vi "Load.vi"(0 "TxA in":T1, 1 "section (optional)":string, 5 "TxO in":T2, 7 "Tx in":T3, 9 "PxA in":T4, 12 "PxO in":T5, 13 "Px in":T6) -> (3 "Px out":T6, 4 "PxO out":T5, 6 "PxA out":T4, 8 "Tx out":T3, 10 "TxO out":T2, 14 "TxA out":T1)   [LabVIEW 2017, in "Konfiguracja.lvlib"]
uses:
  Libraries/Konfiguracja/Konfiguracja.lvlib
  <vilib>/Utility/config.llb/NI_LVConfig.lvlib
  Controls/TxA.ctl
  Controls/TxO.ctl
  Controls/Tx.ctl
  Controls/PxA.ctl
  Controls/Px0.ctl
  Controls/Px.ctl
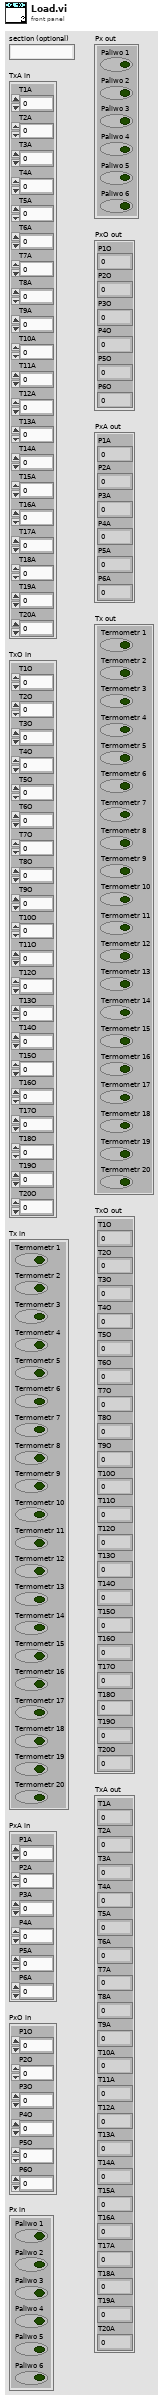
[diagram p1: front panel]
types:
  T1 = typedef "Konfiguracja.lvlib/TxA.ctl" = cluster{"T1A":dbl, "T2A":dbl, "T3A":dbl, "T4A":dbl, "T5A":dbl, "T6A":dbl, "T7A":dbl, "T8A":dbl, "T9A":dbl, "T10A":dbl, "T11A":dbl, "T12A":dbl, "T13A":dbl, "T14A":dbl, "T15A":dbl, "T16A":dbl, "T17A":dbl, "T18A":dbl, "T19A":dbl, "T20A":dbl}
  T2 = typedef "Konfiguracja.lvlib/TxO.ctl" = cluster{"T1O":dbl, "T2O":dbl, "T3O":dbl, "T4O":dbl, "T5O":dbl, "T6O":dbl, "T7O":dbl, "T8O":dbl, "T9O":dbl, "T10O":dbl, "T11O":dbl, "T12O":dbl, "T13O":dbl, "T14O":dbl, "T15O":dbl, "T16O":dbl, "T17O":dbl, "T18O":dbl, "T19O":dbl, "T20O":dbl}
  T3 = typedef "Konfiguracja.lvlib/Tx.ctl" = cluster{"Termometr 1":bool, "Termometr 2":bool, "Termometr 3":bool, "Termometr 4":bool, "Termometr 5":bool, "Termometr 6":bool, "Termometr 7":bool, "Termometr 8":bool, "Termometr 9":bool, "Termometr 10":bool, "Termometr 11":bool, "Termometr 12":bool, "Termometr 13":bool, "Termometr 14":bool, "Termometr 15":bool, "Termometr 16":bool, "Termometr 17":bool, "Termometr 18":bool, "Termometr 19":bool, "Termometr 20":bool}
  T4 = typedef "Konfiguracja.lvlib/PxA.ctl" = cluster{"P1A":dbl, "P2A":dbl, "P3A":dbl, "P4A":dbl, "P5A":dbl, "P6A":dbl}
  T5 = typedef "Konfiguracja.lvlib/Px0.ctl" = cluster{"P1O":dbl, "P2O":dbl, "P3O":dbl, "P4O":dbl, "P5O":dbl, "P6O":dbl}
  T6 = typedef "Konfiguracja.lvlib/Px.ctl" = cluster{"Paliwo 1":bool, "Paliwo 2":bool, "Paliwo 3":bool, "Paliwo 4":bool, "Paliwo 5":bool, "Paliwo 6":bool}
  T7 = typedef "NI_LVConfig.lvlib/Config Data RefNum.ctl" = refnum<k1>
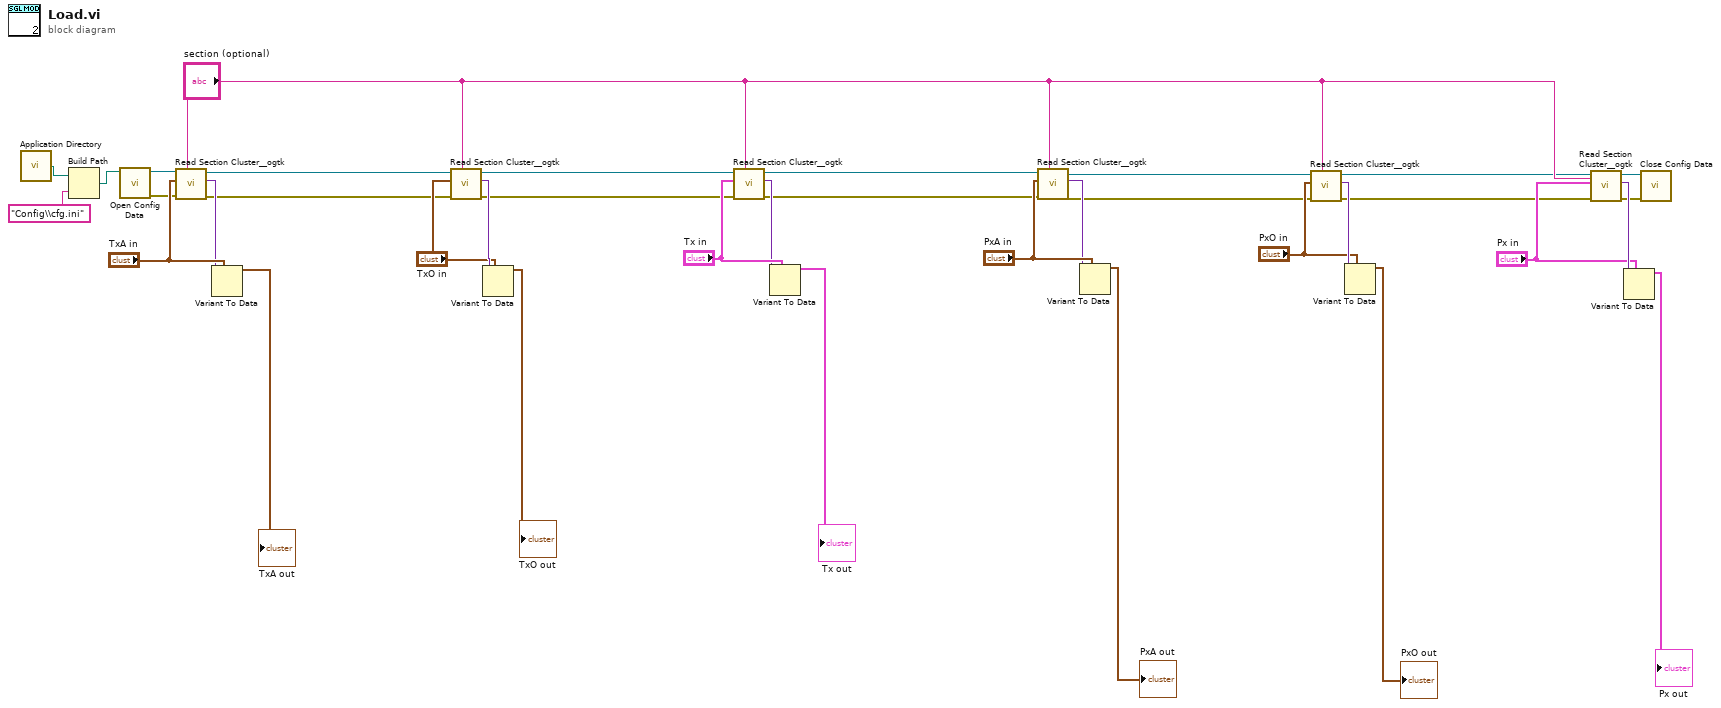
[diagram p0: block diagram]
diagram:
  n1 = call <vilib>:"Application Directory.vi"() -> ("Application Directory"=w1:path)
  n2 = Build Path(base path=w1, name or relative path="Config\\cfg.ini") -> (appended path=w3:path)
  n3 = call <vilib>:"Open Config Data.vi"("configuration file path"=w3) -> ("error out"=w4:errorcluster, "refnum"=w5:T7)  [unwired: 8 in, 1 out]
  n4 = call <userlib>:"Read Section Cluster__ogtk.vi"("section (optional)"="section (optional)", "error in (no error)"=w4, "Section Formatted Cluster Type"="TxA in", "refnum"=w5) -> ("error out"=w6:errorcluster, "Section Formatted Cluster"=w17:variant, "dup refnum"=w7:T7)  [unwired: 3 in, 2 out]
  n5 = Variant To Data(type="TxA in", Variant=w17) -> (data=→"TxA out":T1)  [unwired: 1 in, 1 out]
  n6 = call <userlib>:"Read Section Cluster__ogtk.vi"("section (optional)"="section (optional)", "error in (no error)"=w6, "Section Formatted Cluster Type"="TxO in", "refnum"=w7) -> ("error out"=w8:errorcluster, "Section Formatted Cluster"=w24:variant, "dup refnum"=w9:T7)  [unwired: 3 in, 2 out]
  n7 = Variant To Data(type="TxO in", Variant=w24) -> (data=→"TxO out":T2)  [unwired: 1 in, 1 out]
  n8 = call <userlib>:"Read Section Cluster__ogtk.vi"("section (optional)"="section (optional)", "error in (no error)"=w8, "Section Formatted Cluster Type"="Tx in", "refnum"=w9) -> ("error out"=w10:errorcluster, "Section Formatted Cluster"=w25:variant, "dup refnum"=w11:T7)  [unwired: 3 in, 2 out]
  n9 = Variant To Data(type="Tx in", Variant=w25) -> (data=→"Tx out":T3)  [unwired: 1 in, 1 out]
  n10 = call <userlib>:"Read Section Cluster__ogtk.vi"("section (optional)"="section (optional)", "error in (no error)"=w10, "Section Formatted Cluster Type"="PxA in", "refnum"=w11) -> ("error out"=w12:errorcluster, "Section Formatted Cluster"=w28:variant, "dup refnum"=w13:T7)  [unwired: 3 in, 2 out]
  n11 = Variant To Data(type="PxA in", Variant=w28) -> (data=→"PxA out":T4)  [unwired: 1 in, 1 out]
  n12 = call <userlib>:"Read Section Cluster__ogtk.vi"("section (optional)"="section (optional)", "error in (no error)"=w12, "Section Formatted Cluster Type"="PxO in", "refnum"=w13) -> ("error out"=w14:errorcluster, "Section Formatted Cluster"=w33:variant, "dup refnum"=w15:T7)  [unwired: 3 in, 2 out]
  n13 = Variant To Data(type="PxO in", Variant=w33) -> (data=→"PxO out":T5)  [unwired: 1 in, 1 out]
  n14 = call <userlib>:"Read Section Cluster__ogtk.vi"("section (optional)"="section (optional)", "error in (no error)"=w14, "Section Formatted Cluster Type"="Px in", "refnum"=w15) -> ("error out"=w19:errorcluster, "Section Formatted Cluster"=w36:variant, "dup refnum"=w20:T7)  [unwired: 3 in, 2 out]
  n15 = Variant To Data(type="Px in", Variant=w36) -> (data=→"Px out":T6)  [unwired: 1 in, 1 out]
  n16 = call <vilib>:"Close Config Data.vi"("error in (no error)"=w19, "refnum"=w20) -> ()  [unwired: 8 in, 2 out]
